vi "Build Perimeter Point Array.vi"(11 "Start Point":T2) -> (2 "List No Center Out":T1[](array[typedef]), 3 "No Center Out":T2[](array[typedef]), 5 "With Center Out":T2[](array[typedef]), 7 "List Out":T1[](array[typedef]))   [LabVIEW 2023]
uses:
  Cluster _Point Location.ctl
  ENUM_Location Direction.ctl
  325ebccb-4f04-41cc-a4da-9e6d84605097.vi
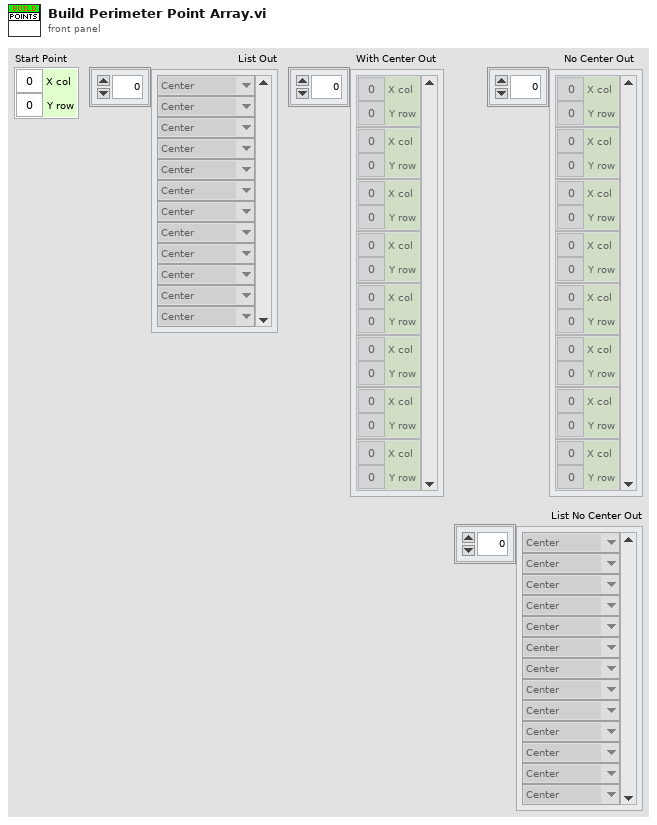
[diagram p1: front panel]
types:
  T1 = typedef "ENUM_Location Direction.ctl" = enum16{"North", "North-East", "East", "South-East", "South", "South-West", "West", "North-West", "Center"}
  T2 = typedef "Cluster _Point Location.ctl" = cluster{"X col":i32, "Y row":i32}
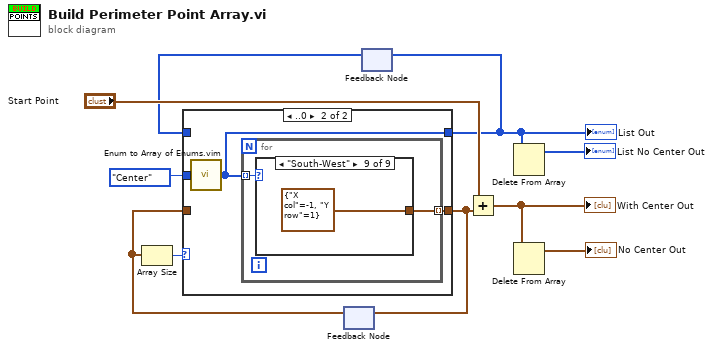
[diagram p0: block diagram]
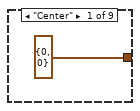
[diagram p3: hidden frame]
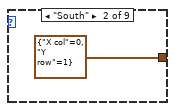
[diagram p4: hidden frame]
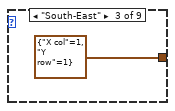
[diagram p5: hidden frame]
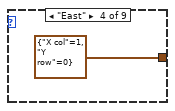
[diagram p6: hidden frame]
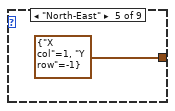
[diagram p7: hidden frame]
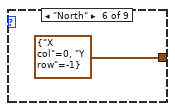
[diagram p8: hidden frame]
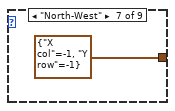
[diagram p9: hidden frame]
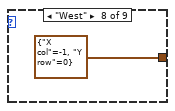
[diagram p10: hidden frame]
diagram:
  n1 = feedback #1() -> (w8:T2[])  [unwired: 1 in]
  n2 = Array Size(array=w8) -> (size(s)=w9:i32)
  n3 = feedback #2() -> (w1:T1[])  [unwired: 1 in]
  n4 = case shown="..0" w9 {
    tunnel: [w12 w15] -> w10
    tunnel: w8 -> [w12 _]
    tunnel: ENUM_Location_Direction."Center" ("Starting Direction") -> [_ w14]
    tunnel: [w11 w13] -> w2
    tunnel: w1 -> [w11 _]
    frame 1.. {
    }
    frame ..0 {
      n5 = call "Enum to Array of Enums.vim"("enum"=w14) -> ("array of enums"=w13:T1[])
      n6 = for {
        tunnel: w13 -> [w17] mode=indexing
        tunnel: [w16] -> w15 mode=indexing
        n7 = case shown="\"South-West\"" w17 {
          tunnel: [T2 {"X col"=0, "Y row"=0} ("Point") T2 {"X col"=0, "Y row"=1} ("Point") T2 {"X col"=1, "Y row"=1} ("Point") T2 {"X col"=1, "Y row"=0} ("Point") T2 {"X col"=1, "Y row"=-1} ("Point") T2 {"X col"=0, "Y row"=-1} ("Point") T2 {"X col"=-1, "Y row"=-1} ("Point") T2 {"X col"=-1, "Y row"=0} ("Point") T2 {"X col"=-1, "Y row"=1} ("Point")] -> w16
          frame "Center" {
          }
          frame "South" {
          }
          frame "South-East" {
          }
          frame "East" {
          }
          frame "North-East" {
          }
          frame "North" {
          }
          frame "North-West" {
          }
          frame "West" {
          }
          frame "South-West" {
          }
        }
      }
    }
  }
  "List Out" <- w2
  n8 = feedback-in #1(w10) -> ()
  n9 = feedback-in #2(w2) -> ()
  n10 = Add(x="Start Point", y=w10) -> (x+y=w5:T2[])
  "With Center Out" <- w5
  n11 = Delete From Array(array=w2) -> (array with subset deleted=→"List No Center Out":T1[])  [unwired: 2 in, 1 out]
  n12 = Delete From Array(array=w5) -> (array with subset deleted=→"No Center Out":T2[])  [unwired: 2 in, 1 out]
